vi "Query Status Register.vi"(8 "error in":errorcluster, 11 "89XX in":refnum<class "89XX.lvclass">) -> (0 "error out":errorcluster, 3 "89XX out":refnum<class "89XX.lvclass">)   [LabVIEW 2019, in "89XX.lvlib" / "89XX.lvclass"]
doc: "Child classes must override this VI:\n\nThis VI is the device specific query of the supply's status registers. \nThe return values are: \n\nThe implementation must read status registers and push the status register values to private data for:\nOCP Flag, OVP Flag, Interlock Flag, Output Flag into the private data arrays of the power supply class."
uses:
  Library/89XX.lvclass
  C:/Users/Public/Documents/Development/builds/Instruments/PowerSupply.lvlibp/Library/PowerSupply.lvclass
  builds/Instruments/PowerSupply.lvlibp/Custom Controls/Status_Flags.ctl
  builds/Instruments/PowerSupply.lvlibp/Accessors/Write Status Flags.vi
  builds/Instruments/PowerSupply.lvlibp/Library/PowerSupply.lvclass
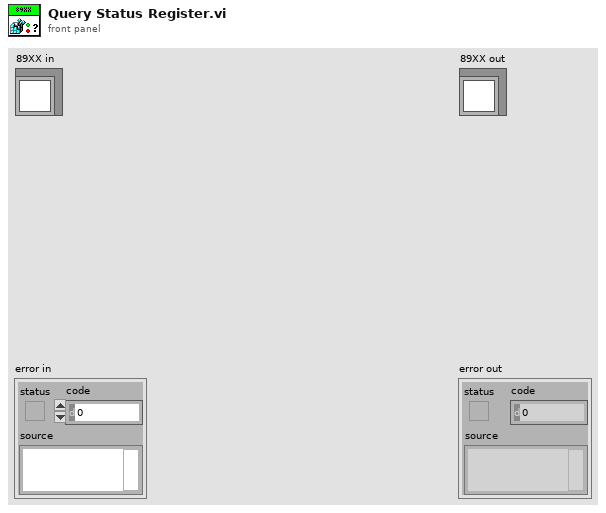
[diagram p1: front panel]
types:
  T1 = typedef "PowerSupply.lvlibp/PowerSupply.lvclass/Status_Flags.ctl" = cluster{"Interlock":bool, "OVP":bool, "OCP":bool, "Output":bool}
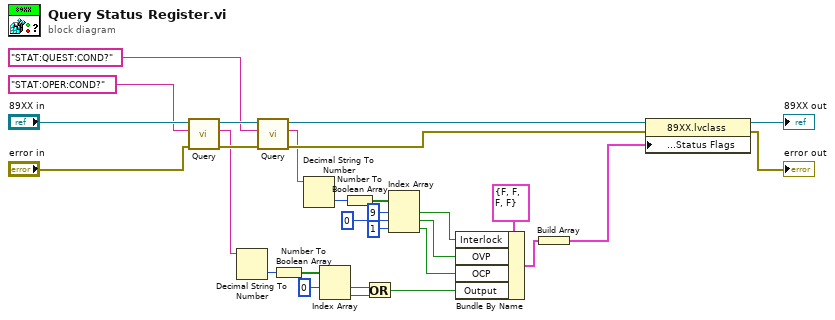
[diagram p0: block diagram]
diagram:
  n1 = call "Query.vi"("error in"="error in", "Query"="STAT:OPER:COND?", "89XX in"="89XX in") -> ("error out"=w25:errorcluster, "Response"=w20:string, "89XX out"=w29:refnum<class "89XX.lvclass">)  [unwired: 6 in]
  n2 = Decimal String To Number(string=w20) -> (number=w14:i32)  [unwired: 2 in, 1 out]
  n3 = call "Query.vi"("error in"=w25, "Query"="STAT:QUEST:COND?", "89XX in"=w29) -> ("error out"=w23:errorcluster, "Response"=w19:string, "89XX out"=w26:refnum<class "89XX.lvclass">)  [unwired: 6 in]
  n4 = Number To Boolean Array(number=w14) -> (Boolean array=w12:bool[])
  n5 = Decimal String To Number(string=w19) -> (number=w13:i32)  [unwired: 2 in, 1 out]
  n6 = Index Array(array=w12, index #1=0 ("index")) -> (element #1=w3:bool, element #2=w4:bool)  [unwired: 1 in]
  n7 = Number To Boolean Array(number=w13) -> (Boolean array=w11:bool[])
  n8 = Or(x=w3, y=w4) -> (x .or. y?=w2:bool)
  n9 = Index Array(array=w11, index #1=9 ("index"), index #2=0 ("index"), index #3=1 ("index")) -> (element #1=w9:bool, element #2=w8:bool, element #3=w7:bool)
  n10 = Bundle By Name(cluster=T1 {"Interlock"=FALSE, "OVP"=FALSE, "OCP"=FALSE, "Output"=FALSE} ("Status"), "Interlock"=w9, "OVP"=w8, "OCP"=w7, "Output"=w2) -> (w17:T1)
  n11 = Build Array(w17) -> (w15:T1[])
  n12 = property class="89XX.lvclass"(reference=w26, error in=w23, "Accessors:GUI:Status:Status Flags"=w15) -> (reference out=→"89XX out":refnum<class "89XX.lvclass">, error out=→"error out":errorcluster)
